vi "AA_clearing.vi"(0 "Archivo de\nreferencias (.csv)":path, 4 "FEATS":path, 5 "ARCHIVO\nTDMS":path, 7 "Largo de ventada temporal en N samples":dbl=44100.0, 9 "Canal":string[](array[string])=["Sound Pressure_0"], 11 "frequency range":T2={"low band"=enum."20 Hz", "high band"=enum."20000 Hz"}) -> ()   [LabVIEW 2017]
uses:
  <vilib>/Waveform/WDTOps.llb/WDT Get Waveform Subset DBL.vi
  <vilib>/addons/Sound and Vibration/svt_Octave_2014 standard/SVT Third-octave Analysis (1 Ch).vi
  <vilib>/addons/Sound and Vibration/svt_Octave_2014 standard/SVT Weighting Filter (octave) (1 Ch).vi
  <vilib>/addons/Sound and Vibration/svt_Level/SVT Sound Level (1 Ch).vi
  <vilib>/Utility/file.llb/Write Delimited Spreadsheet (string).vi
  <vilib>/addons/Sound and Vibration/svt_Octave/SoundVib_Octave_2014 standard.lvlib
  <vilib>/addons/Sound and Vibration/svt_Level/SoundVib_SoundLevel.lvlib
panel:
  out "# obs\nBands":i32[](array[numeric])
  out "# obs\nLevels A":i32
  out "current\nLevel A":dbl format="%.2f"
  in  "restart L_bands":bool=TRUE
  out "Multiplot \noctave graph 2":T1(graph)
  out "Levels_lineal":dbl[](array[numeric])
  out "Para el CSV, excepto fecha y hora":string[][](array[string])
  out "TO CSV.":string[][](array[string])
  out "ETIQUETAS":string[](array[string])
  out "BANDAS":dbl[][](array[numeric])
  out "Samples \npor Objeto":waveform(dbl)
  out "Secciones":waveform(dbl)[](array[waveform])
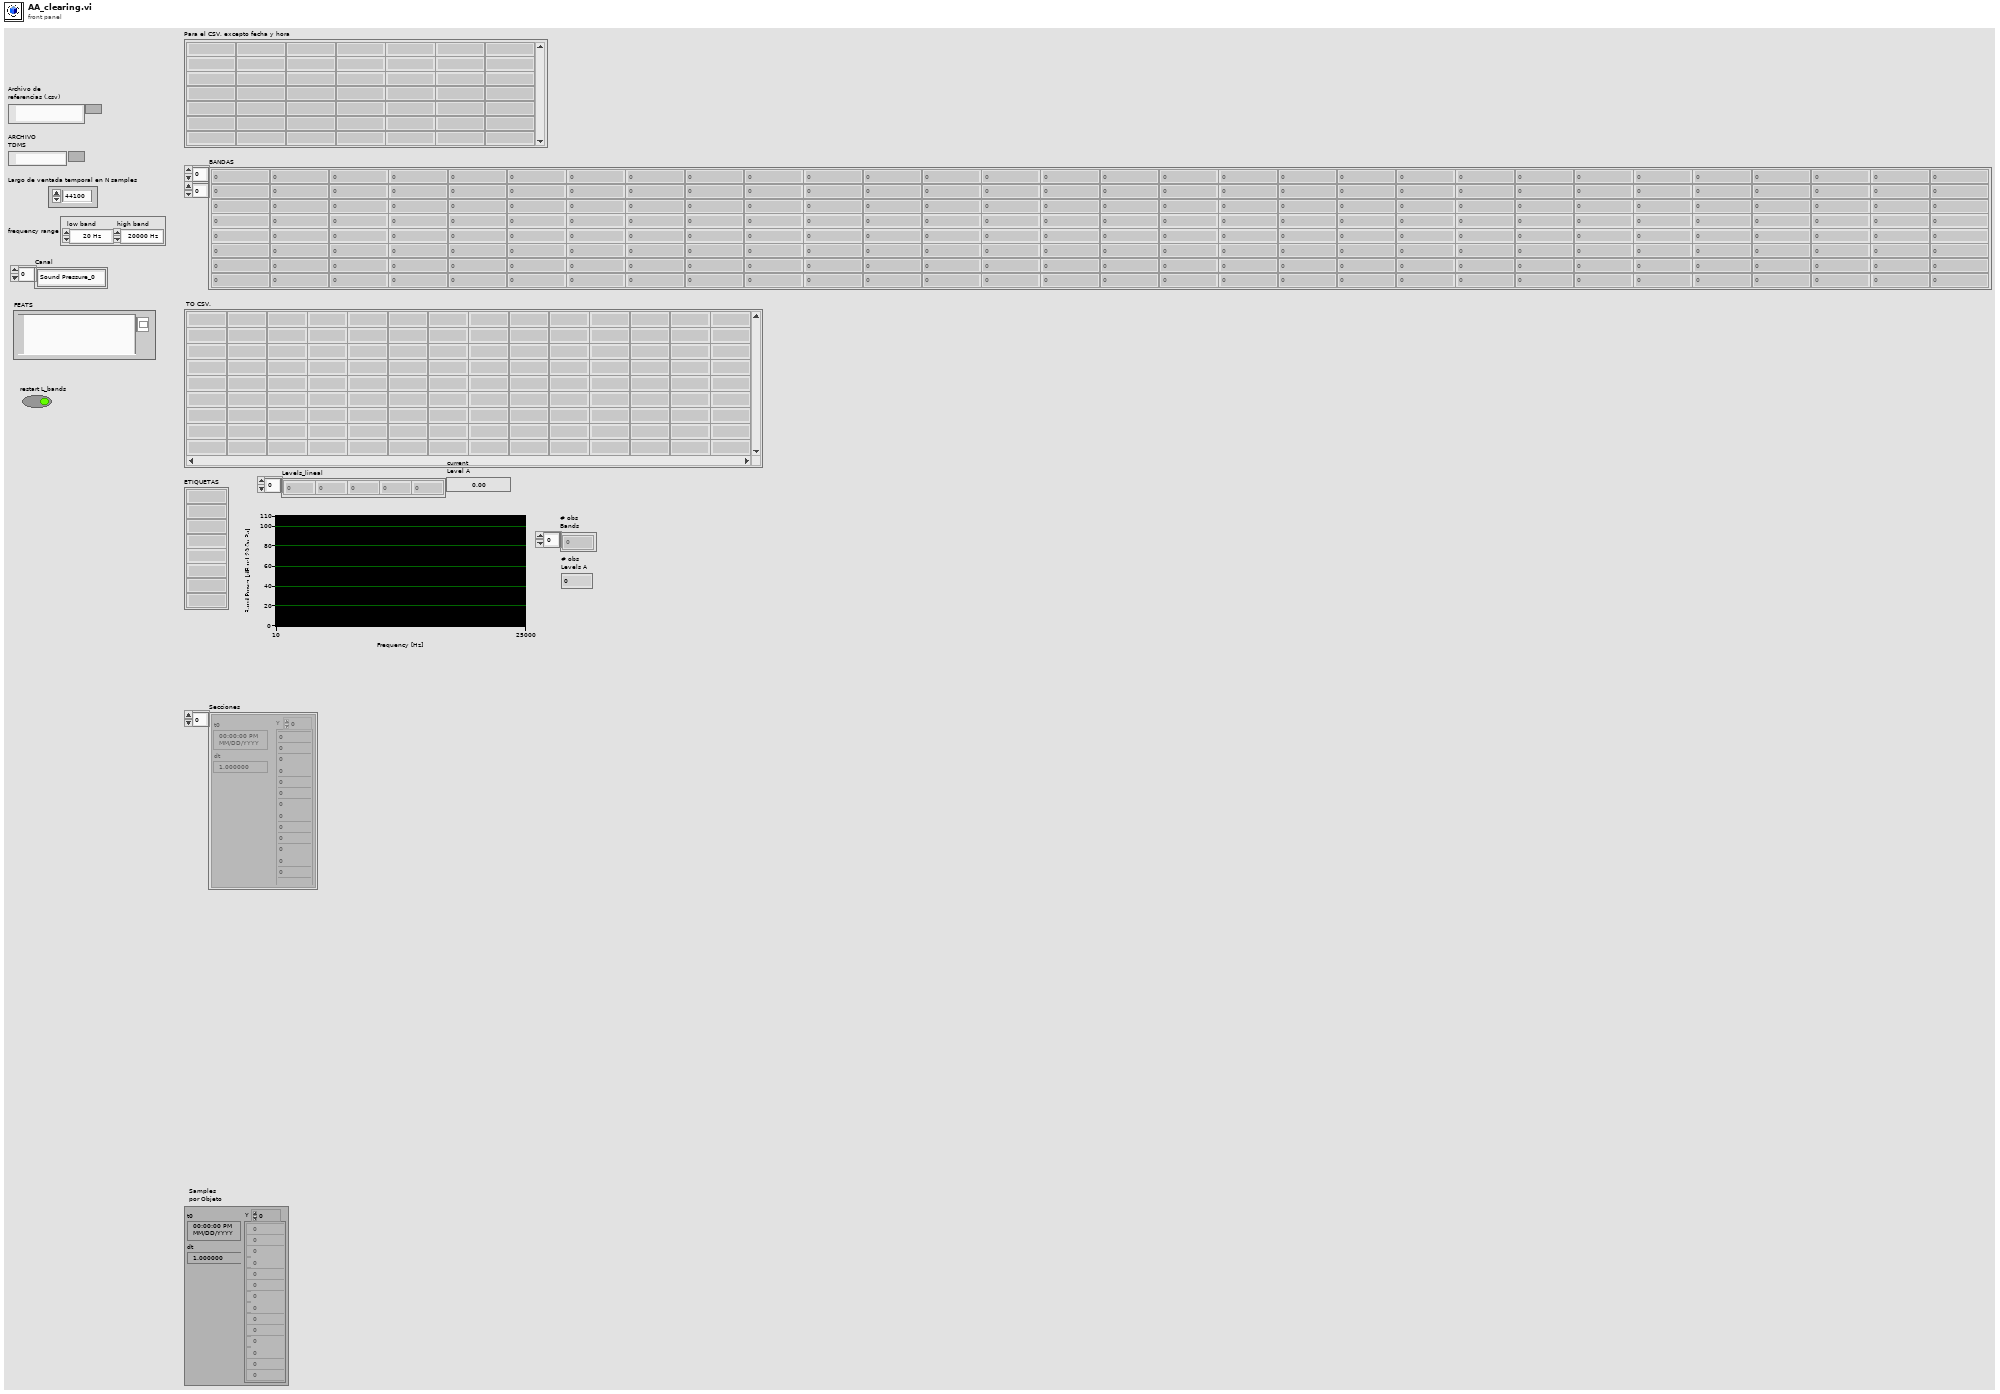
[diagram p1: front panel]
types:
  T1 = cluster{"nominal frequencies [Hz]":dbl[], "band power":dbl[]}
  T2 = cluster{"low band":enum16{"20 Hz", "25 Hz", "31.5 Hz", "40 Hz", "50 Hz", "63 Hz", "80 Hz", "100 Hz", "125 Hz", "160 Hz", "200 Hz", "250 Hz", "315 Hz", "400 Hz", "500 Hz", "630 Hz", "800 Hz", "1000 Hz", "1250 Hz", "1600 Hz", "2000 Hz", "2500 Hz", "3150 Hz", "4000 Hz", "5000 Hz", "6300 Hz", "8000 Hz", "10000 Hz", "12500 Hz", "16000 Hz", "20000 Hz"}, "high band":enum16{"20 Hz", "25 Hz", "31.5 Hz", "40 Hz", "50 Hz", "63 Hz", "80 Hz", "100 Hz", "125 Hz", "160 Hz", "200 Hz", "250 Hz", "315 Hz", "400 Hz", "500 Hz", "630 Hz", "800 Hz", "1000 Hz", "1250 Hz", "1600 Hz", "2000 Hz", "2500 Hz", "3150 Hz", "4000 Hz", "5000 Hz", "6300 Hz", "8000 Hz", "10000 Hz", "12500 Hz", "16000 Hz", "20000 Hz"}}
  T3 = enum16{"open", "open or create", "create or replace", "create", "open (read-only)"}
  T4 = enum16{"Linear", "Exponential", "Equal confidence", "Peak"}
  T5 = cluster{"Leq":bool, "Running Leq":bool, "Exponential":bool, "Peak":bool}
  T6 = typedef "svc_Octave Info.ctl" = cluster{"standard":T7, "bandwidth":enum16{"1 octave", "1/3 octave", "1/6 octave", "1/12 octave", "1/24 octave"}, "low band":i32, "high band":i32, "weighting filter":T8, "dB reference":dbl, "dB On":bool, "unit label":string, "channel name":string, "description":string, "engineering units":T9, "custom label":string, "spectrum type":enum16{"power", "magnitude"}, "spectral density":bool, "filters settled":bool}
  T7 = typedef "svc_Octave Standard.ctl" = enum16{"ANSI S1.11", "IEC 61260"}
  T8 = typedef "svc_Weighting Filter Text Ring.ctl" = u16
  T9 = typedef "svc_Engineering Units Text Ring.ctl" = u16
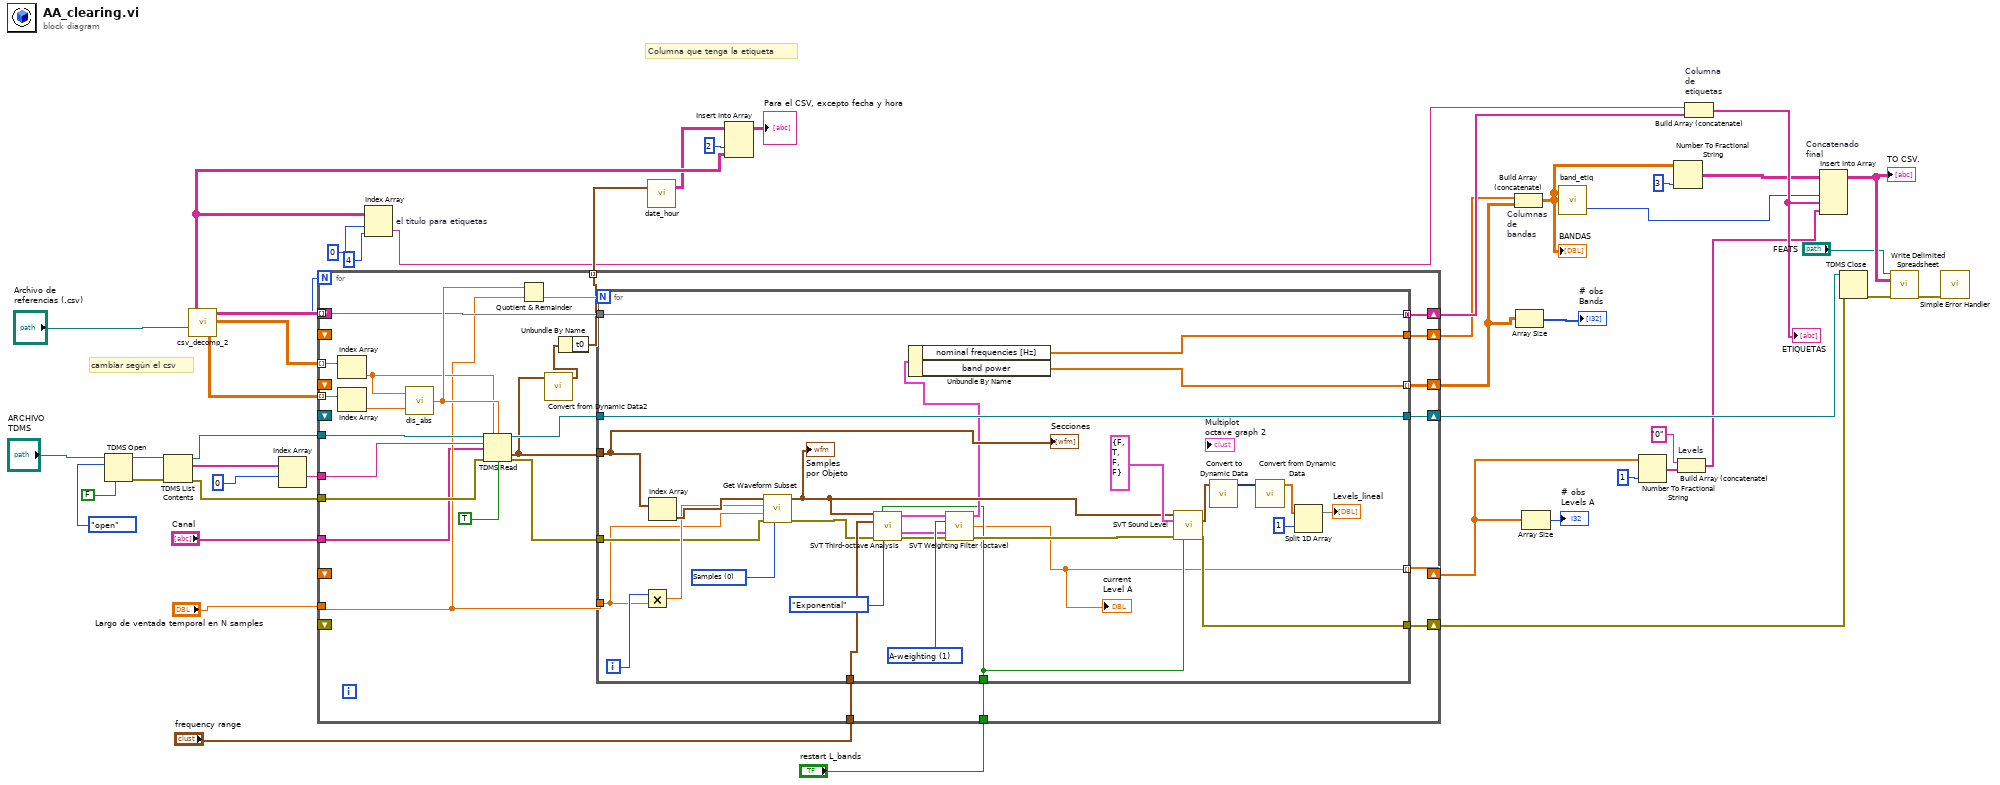
[diagram p0: block diagram]
diagram:
  # "cambiar según el csv"
  # "Columna que tenga la etiqueta"
  n1 = TDMS Open(6:FALSE ("disable buffering? (T)"), 10:T3."open" ("operation (0:open)"), 11:"ARCHIVO\nTDMS") -> (0:w16:errorcluster, 3:w38:refnum<k34>)  [unwired: 4 in]
  n2 = TDMS List Contents(4:w16, 7:w38) -> (0:w40:errorcluster, 2:w39:string[], 3:w17:refnum<k34>)  [unwired: 1 in, 1 out]
  n3 = call "csv_decomp_2.vi"("Archivo de referencias (.csv)"="Archivo de\nreferencias (.csv)") -> ("finales"=w44:dbl[][], "iniciales"=w45:dbl[][], "etiquetas"=w43:string[][], "# dimención"=w10:i32, "Lectura CSV"=w41:string[][])  [unwired: 2 in]
  n4 = Index Array(array=w39, index #1=0 ("index")) -> (element #1=w19:string)  [unwired: 1 in, 1 out]
  n5 = for {
    N: w10 -> [_]
    tunnel: w45 -> [w71] mode=indexing
    tunnel: w44 -> [w72] mode=indexing
    tunnel: w43 -> [w60] mode=indexing
    tunnel: w17 -> [w73]
    tunnel: w40 -> [w66]
    tunnel: w19 -> [w74]
    tunnel: "Largo de ventada temporal en N samples" -> [w56]
    tunnel: [w53] -> w34 mode=indexing
    tunnel: "Canal" -> [w51]
    tunnel: "frequency range" -> [w50]
    tunnel: "restart L_bands" -> [w49]
    shift-right: [w52] -> w4
    shift-left: _ -> [_]
    shift-right: [w64] -> w20
    shift-left: _ -> [_]
    shift-right: [w59] -> w25
    shift-left: _ -> [_]
    shift-right: [w63] -> w21
    shift-left: _ -> [_]
    shift-right: [w62] -> w6
    shift-left: _ -> [_]
    shift-right: [w61] -> w8
    shift-left: _ -> [_]
    n6 = Index Array(array=w71) -> (element=w58:dbl)  [unwired: 1 in]
    n7 = Index Array(array=w72) -> (element=w57:dbl)  [unwired: 1 in]
    n8 = call "dis_abs.vi"("Numeric in"=w57, "Numeric 3"=w58) -> ("distancia abs entre dos números"=w67:dbl)
    n9 = TDMS Read(0:w73, 1:w58, 2:w67, 5:w74, 7:w51, 11:w66, 13:TRUE ("return channels in file order? (F)")) -> (4:w70:refnum<k34>, 10:w55:waveform(dbl)[], 15:w65:errorcluster)  [unwired: 1 in, 3 out]
    n10 = Quotient & Remainder(x=w67, y=w56) -> (floor(x/y)=w68:dbl)  [unwired: 1 out]
    n11 = call "Convert from Dynamic Data2"("Dynamic Data Type"=w55) -> ("Waveform"=w54:waveform(dbl))  [unwired: 3 in]
    n12 = Unbundle By Name(w54) -> ("t0"=w53:timestamp)
    n13 = for {
      N: w68 -> [_]
      tunnel: w70 -> [w100]
      tunnel: w55 -> [w94]
      tunnel: w65 -> [w101]
      tunnel: [w93] -> w61
      tunnel: [w100] -> w64
      tunnel: [w99] -> w63
      tunnel: [w98] -> w62 mode=indexing
      tunnel: w60 -> [w97]
      tunnel: [w97] -> w59 mode=concatenating
      tunnel: w56 -> [w95]
      tunnel: [w75] -> w52 mode=indexing
      tunnel: w50 -> [w92]
      tunnel: w49 -> [w77]
      i -> [w96]
      w83 = u16 1 items=["Linear", "A-weighting", "B-weighting", "C-weighting"] ("weighting")
      w103 = u16 0 items=["Samples", "Relative Time"] ("start/duration format")
      n14 = Multiply(x=w96, y=w95) -> (x*y=w102:dbl)
      n15 = Index Array(array=w94) -> (element=w104:waveform(dbl))  [unwired: 1 in]
      n16 = call-poly <vilib>:"Get Waveform Subset.vi"("start/duration format"=w103, "error in (no error)"=w101, "duration"=w95, "start samples/time"=w102, "waveform in"=w104) -> ("error out"=w85:errorcluster, "waveform out"=w86:waveform(dbl))  [unwired: 1 in, 2 out]
      "Samples \npor Objeto" <- w86
      n17 = call-poly <vilib>:"SVT Third-octave Analysis.vi"("scaled signal [EU]"=w86, "restart averaging (F)"=w77, "frequency range"=w92, "error in (no error)"=w85, "averaging type"=T4."Exponential") -> ("octave spectrum"=w84:T1, "octave info"=w79:T6, "error out"=w81:errorcluster)  [unwired: 5 in, 3 out]
      n18 = call-poly <vilib>:"SVT Weighting Filter (octave).vi"("octave spectrum"=w84, "weighting"=w83, "octave info in"=w79, "error in (no error)"=w81) -> ("weighted octave spectrum"=w82:T1, "total band power"=w75:dbl, "error out"=w80:errorcluster)  [unwired: 7 in, 2 out]
      "current\nLevel A" <- w75
      n19 = Unbundle By Name(w82) -> ("nominal frequencies [Hz]"=w99:dbl[], "band power"=w98:dbl[])
      n20 = call-poly <vilib>:"SVT Sound Level.vi"("scaled signal [EU]"=w86, "measurement selection"=T5 {"Leq"=FALSE, "Running Leq"=TRUE, "Exponential"=FALSE, "Peak"=FALSE}, "error in (no error)"=w80, "restart averaging (F)"=w77) -> ("running Leq sound level [dB EU]"=w76:waveform(dbl), "error out"=w93:errorcluster)  [unwired: 6 in, 4 out]
      n21 = call "Convert to Dynamic Data"("Array"=w76) -> ("Dynamic Data Type"=w87:dynamicdata)  [unwired: 3 in]
      n22 = call "Convert from Dynamic Data"("Dynamic Data Type"=w87) -> ("Array"=w90:dbl[])  [unwired: 3 in]
      n23 = Split 1D Array(array=w90, index=1) -> (first subarray=→"Levels_lineal":dbl[])  [unwired: 1 out]
      "Secciones" <- w94
    }
  }
  n24 = Index Array "el título para etiquetas"(array=w41, index (row)=0 ("disabled index (row)"), index (col)=4 ("disabled index (col)")) -> (element=w28:string)
  n25 = call "date_hour.vi"("Array"=w34) -> ("appended array"=w35:string[][])  [unwired: 1 in, 1 out]
  n26 = Insert Into Array(array=w35, index (col)=2 ("disabled index (col)"), new element=w41) -> (→"Para el CSV, excepto fecha y hora":string[][])  [unwired: 1 in]
  n27 = Build Array (concatenate) "Columnas \nde\nbandas"(w21, w6) -> (w31:dbl[][])
  "BANDAS" <- w31
  n28 = Array Size(array=w6) -> (size(s)=→"# obs\nBands":i32[])
  n29 = Array Size(array=w4) -> (size(s)=→"# obs\nLevels A":i32)
  n30 = call "band_etiq.vi"("Array de entrada"=w31) -> ("Numeric"=w32:i32)  [unwired: 1 in, 1 out]
  n31 = Number To Fractional String(number=w4, precision (6)=i16 1) -> (F-format string=w2:string[])  [unwired: 2 in]
  n32 = Number To Fractional String(number=w31, precision (6)=i16 3) -> (F-format string=w30:string[][])  [unwired: 2 in]
  n33 = Build Array (concatenate) "Levels"("0", w2) -> (w1:string[])
  n34 = Build Array (concatenate) "Columna \nde \netiquetas"(w28, w25) -> (w48:string[])
  "ETIQUETAS" <- w48
  n35 = Insert Into Array "Concatenado \nfinal"(array=w30, index (col)=w32, new element #1=w48, new element #2=w1) -> (w47:string[][])  [unwired: 1 in]
  "TO CSV." <- w47
  n36 = TDMS Close(8:w8, 11:w20) -> (0:w23:errorcluster)  [unwired: 1 out]
  n37 = call-poly <vilib>:"Write Delimited Spreadsheet.vi"("file path (dialog if empty)"="FEATS", "2D data"=w47, "error in (no error)"=w23) -> ("error out"=w24:errorcluster)  [unwired: 11 in, 1 out]
  n38 = call <vilib>:"Simple Error Handler.vi"("error in (no error)"=w24) -> ()  [unwired: 4 in, 5 out]
